vi "p6100_write.vi"(0 "VISA in":refnum<visa-resource-name>, 1 "Serial Parameters":T1, 2 "Setpoint":cluster{u8, u8}, 3 "error in":errorcluster) -> (5 "VISA out":refnum<visa-resource-name>, 6 "Temp":cluster{"Bottom":dbl, "Top":dbl}, 7 "error out":errorcluster)   [LabVIEW 2011]
uses:
  <vilib>/NI Modbus.llb/MB Serial Master Query Write Single Register (poly).vi
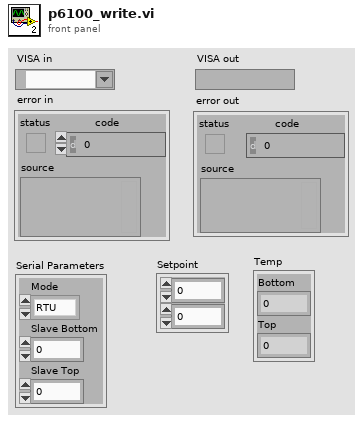
[diagram p1: front panel]
types:
  T1 = cluster{"Mode":enum16{"RTU", "ASCII"}, "Slave Bottom":u8, "Slave Top":u8}
  T2 = cluster{"Mode":enum16{"RTU", "ASCII"}, "Slave Bottom":u8}
  T3 = cluster{"Mode":enum16{"RTU", "ASCII"}, "Slave Top":u8}
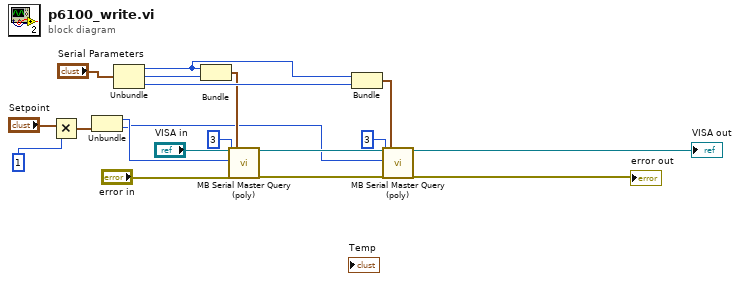
[diagram p0: block diagram]
diagram:
  n1 = Multiply(x="Setpoint", y=u8 1) -> (x*y=w7:cluster{u8, u8})
  n2 = Unbundle(w7) -> (w4:u8, w3:u8)
  n3 = Unbundle("Serial Parameters") -> ("Mode"=w12:enum16{"RTU", "ASCII"}, "Slave Bottom"=w14:u8, "Slave Top"=w13:u8)
  n4 = Bundle("Mode"=w12, "Slave Bottom"=w14) -> (w11:T2)  [unwired: 1 in]
  n5 = call-poly <vilib>:"MB Serial Master Query (poly).vi"("VISA resource name"="VISA in", "Address"=u16 3, "Holding Register"=w4, "error in"="error in", "Serial Parameters"=w11) -> ("VISA resource name out"=w19:refnum<visa-resource-name>, "error out"=w18:errorcluster)  [unwired: 12 in, 1 out]
  n6 = Bundle("Mode"=w12, "Slave Top"=w13) -> (w10:T3)  [unwired: 1 in]
  n7 = call-poly <vilib>:"MB Serial Master Query (poly).vi"("VISA resource name"=w19, "Address"=u16 3, "Holding Register"=w3, "error in"=w18, "Serial Parameters"=w10) -> ("VISA resource name out"=→"VISA out":refnum<visa-resource-name>, "error out"=→"error out":errorcluster)  [unwired: 12 in, 1 out]
